vi "Get Historc MC List Box View VI Ref.vi"(8 "error in (no error)":errorcluster, 11 "Messages Composite View In":refnum<class "Messages Composite View.lvclass">) -> (0 "error out":errorcluster, 2 "VI Ref":refnum<vi>, 3 "Messages Composite View Out":refnum<class "Messages Composite View.lvclass">)   [LabVIEW 2020, in "Messages Composite View.lvclass"]
uses:
  Messages Composite View.lvclass
  Messages Composite View.lvclass/Messages Composite View.ctl
  Debug View/Debug View.lvclass/Debug View.ctl
  Debug View/Debug View.lvclass
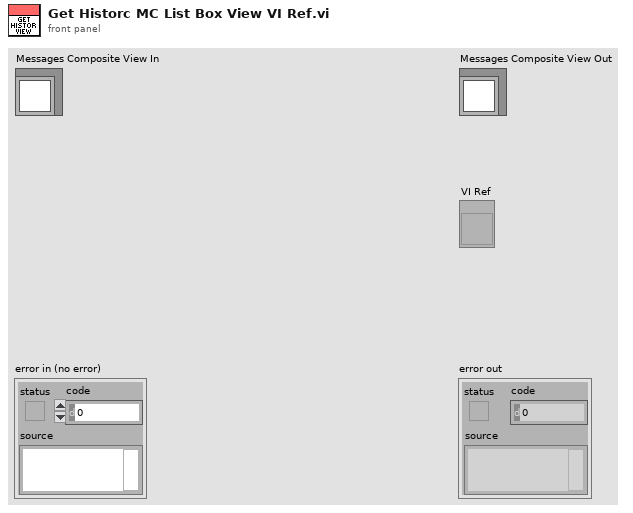
[diagram p1: front panel]
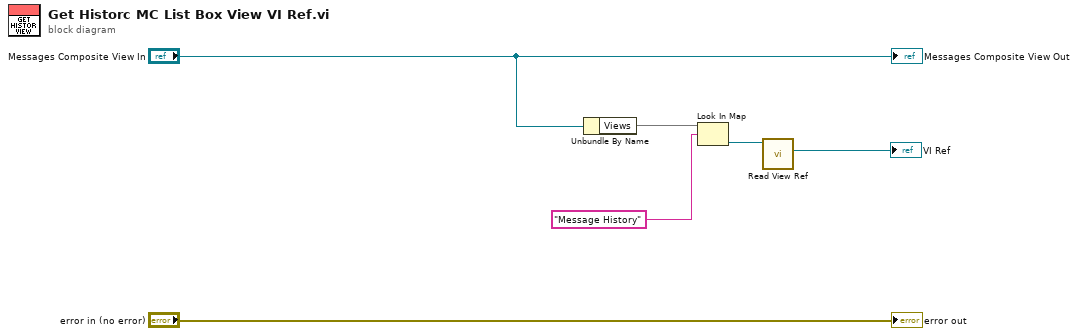
[diagram p0: block diagram]
diagram:
  n1 = Unbundle By Name("Messages Composite View In") -> ("Views"=w4:map{string, refnum<class "Debug View.lvclass">})
  n2 = Look In Map(map=w4, key="Message History" ("Name")) -> (value=w2:refnum<class "Debug View.lvclass">)  [unwired: 1 in, 1 out]
  n3 = call "Read View Ref.vi"("Debug View In"=w2) -> ("View Ref"=→"VI Ref":refnum<vi>)  [unwired: 8 in, 2 out]
  "error out" <- "error in (no error)"
  "Messages Composite View Out" <- "Messages Composite View In"
